vi "Rx GlobalStat to DBLs.vi"(11 "Rx GlobalStat in":T1={"TotalByteCount"=[0], "FrameGoodCount"=[0], "FrameErrorCount"=[0], "BytesPerSecond"=[0], "FramesPerSecond"=[0], "PhysErrorCount"=[0], "PreamErrorCount"=[0], "UnaligErrorCount"=[0], "CRCErrorCount"=[0], "IFGErrorCount"=[0], "IPErrorCount"=[0], "MACErrorCount"=[0], "NoSfdErrorCount"=[0], "VLLenErrorCount"=[0], "SNIntegrityErrorCount"=[0], "TrafShapingViolationCount"=[0], "MAC1Short"=[0], "MAC64To127Count"=[0], "MAC128To255Count"=[0], "MAC256To511Count"=[0], "MAC512To1023Count"=[0], "MAC1024To1518Count"=[0], "MACLong"=[0]}) -> (3 "Rx GlobalStat DBL Array":dbl[](array[numeric]))   [LabVIEW 2020, in "afdx_custom_device Engine.lvlib" / "Implementation.lvlib" / "Monitor Execution Unit.lvclass"]
uses:
  Monitor Execution Unit.lvclass
  AIM LabVIEW src/src/AIM664LV.lvlib
  afdx_custom_device Engine.lvlib
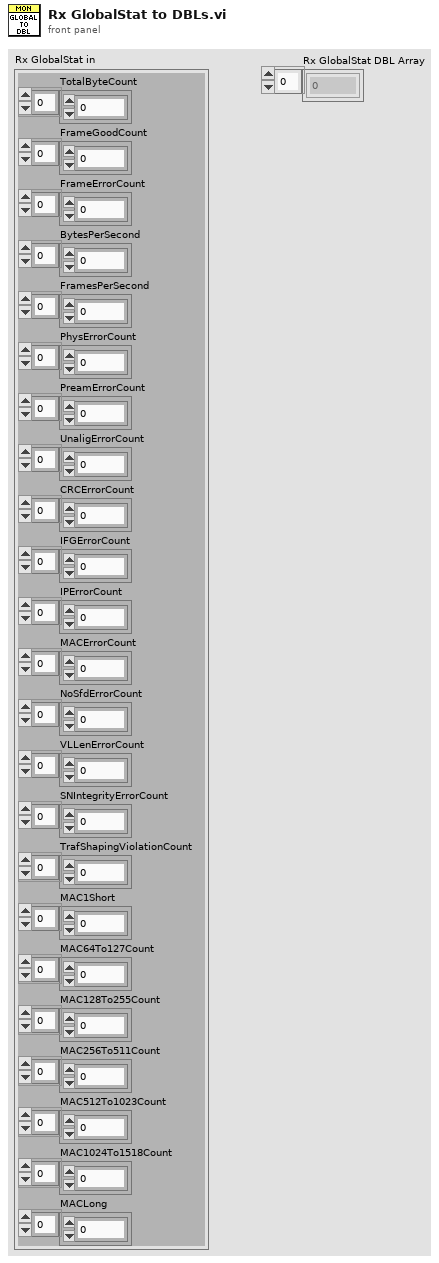
[diagram p1: front panel]
types:
  T1 = cluster{"TotalByteCount":u32[], "FrameGoodCount":u32[], "FrameErrorCount":u32[], "BytesPerSecond":u32[], "FramesPerSecond":u32[], "PhysErrorCount":u32[], "PreamErrorCount":u32[], "UnaligErrorCount":u32[], "CRCErrorCount":u32[], "IFGErrorCount":u32[], "IPErrorCount":u32[], "MACErrorCount":u32[], "NoSfdErrorCount":u32[], "VLLenErrorCount":u32[], "SNIntegrityErrorCount":u32[], "TrafShapingViolationCount":u32[], "MAC1Short":u32[], "MAC64To127Count":u32[], "MAC128To255Count":u32[], "MAC256To511Count":u32[], "MAC512To1023Count":u32[], "MAC1024To1518Count":u32[], "MACLong":u32[]}
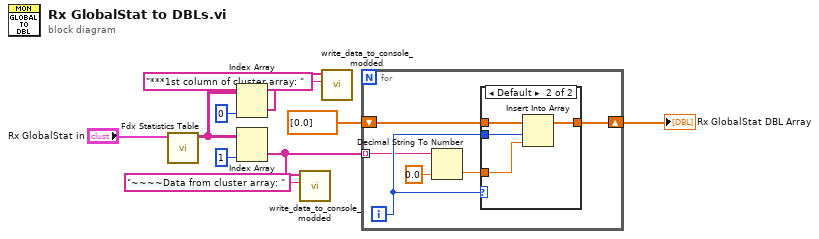
[diagram p0: block diagram]
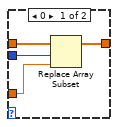
[diagram p2: hidden frame]
diagram:
  n1 = call "Fdx Statistics Table.vi"("GlobalStat Out"="Rx GlobalStat in") -> ("Table Control"=w4:string[][])  [unwired: 10 in]
  n2 = Index Array(array=w4, index (col)=0 ("disabled index (col)")) -> (element=w2:string[])  [unwired: 1 in]
  n3 = Index Array(array=w4, index (col)=1 ("disabled index (col)")) -> (element=w9:string[])  [unwired: 1 in]
  n4 = call "write_data_to_console_modded.vi"("Tag"="~~~~Data from cluster array: ", "Data"=w9) -> ()  [unwired: 9 in, 1 out]
  n5 = call "write_data_to_console_modded.vi"("Tag"="***1st column of cluster array: ", "Data"=w2) -> ()  [unwired: 9 in, 1 out]
  n6 = for {
    tunnel: w9 -> [w12] mode=indexing
    shift-right: [w15] -> w7
    shift-left: dbl[] [0.0] -> [w16]
    i -> [w14]
    n7 = Decimal String To Number(string=w12, default (0L)=0.0 ("default (0 I32)")) -> (number=w11:dbl)  [unwired: 1 in, 1 out]
    n8 = case shown="Default" w14 {
      tunnel: w16 -> [w20 w24]
      tunnel: w14 -> [w17 w23]
      tunnel: [w19 w22] -> w15
      tunnel: w11 -> [w18 w21]
      frame 0 {
        n9 = Replace Array Subset(array=w20, new element=w18, index=w17) -> (w19:dbl[])
      }
      frame Default {
        n10 = Insert Into Array(array=w24, index=w23, new element=w21) -> (w22:dbl[])
      }
    }
  }
  "Rx GlobalStat DBL Array" <- w7
